vi "OphirClose.vi"(0 "OphirPM":T1, 5 "error in":errorcluster) -> (19 "error out":errorcluster)   [LabVIEW 2012]
panel:
  # "OPHIR USBI Close"
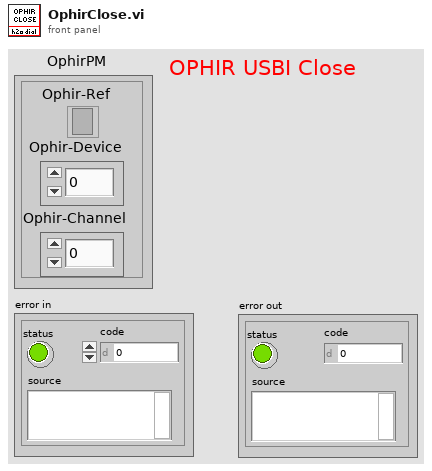
[diagram p1: front panel]
types:
  T1 = cluster{"Ophir-Ref":refnum<k7>, "Ophir-Device":i32, "Ophir-Channel":i32}
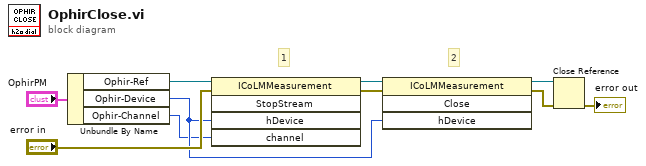
[diagram p0: block diagram]
diagram:
  # "2"
  # "1"
  n1 = Unbundle By Name("OphirPM") -> ("Ophir-Ref"=w3:refnum<k7>, "Ophir-Device"=w2:i32, "Ophir-Channel"=w1:i32)
  n2 = invoke class="ICoLMMeasurement" method="StopStream"(reference=w3, error in="error in", "hDevice"=w2, "channel"=w1) -> (reference out=w7:refnum<k7>, error out=w6:errorcluster)  [unwired: 1 in, 3 out]
  n3 = invoke class="ICoLMMeasurement" method="Close"(reference=w7, error in=w6, "hDevice"=w2) -> (reference out=w10:refnum<k7>, error out=w9:errorcluster)  [unwired: 1 in, 2 out]
  n4 = Close Reference(reference=w10, error in (no error)=w9) -> (error out=→"error out":errorcluster)
